vi "SetPin.vi"(0 "Cypress CY8CKIT-059 in":refnum<class "Cypress CY8CKIT-059.lvclass">, 5 "Port":u8, 7 "Pin":u8, 9 "Value":bool, 11 "error in (no error)":errorcluster) -> (4 "Cypress CY8CKIT-059 out":refnum<class "Cypress CY8CKIT-059.lvclass">, 15 "error out":errorcluster)   [LabVIEW 2020, in "Cypress CY8CKIT-059.lvclass"]
doc: "Sends a command to write on a pin of the target device."
uses:
  Cypress CY8CKIT-059.lvclass
  MCU/MCU.lvclass
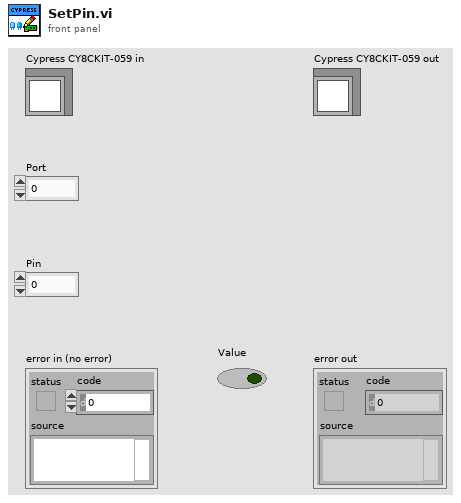
[diagram p1: front panel]
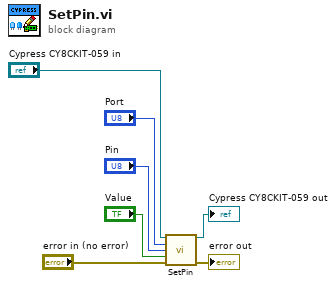
[diagram p0: block diagram]
diagram:
  n1 = call-parent "SetPin.vi"("MCU in"="Cypress CY8CKIT-059 in", "Port"="Port", "Pin"="Pin", "Value"="Value", "error in (no error)"="error in (no error)") -> ("MCU out"=→"Cypress CY8CKIT-059 out":refnum<class "Cypress CY8CKIT-059.lvclass">, "error out"=→"error out":errorcluster)  [unwired: 9 in]
